vi "test_Template.vi"(8 "error in":errorcluster, 9 "tear down connection":bool, 10 "set-up a connection":bool, 11 "device selection":enum16{"monochromator", "CCD", "SCD"}(ring)) -> (0 "error out":errorcluster)   [LabVIEW 2023]
uses:
  Source/Classes/CCD/CCD.lvclass
  <vilib>/addons/_JKI Toolkits/Caraya/classes/Assert/Assert Not Error.vi
  <vilib>/addons/_JKI Toolkits/Caraya/classes/Assert/Assert Equal Value_Variant.vi
  Source/Classes/GenericDevice/GenericDevice.lvclass
  <vilib>/addons/_JKI Toolkits/Caraya/classes/Test/Test.lvclass
  <vilib>/addons/_JKI Toolkits/Caraya/classes/Assert/Assert.lvclass
panel:
  # "Connector Pane"
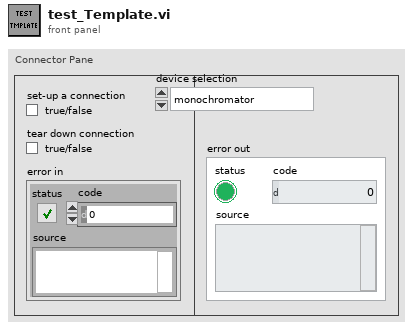
[diagram p1: front panel]
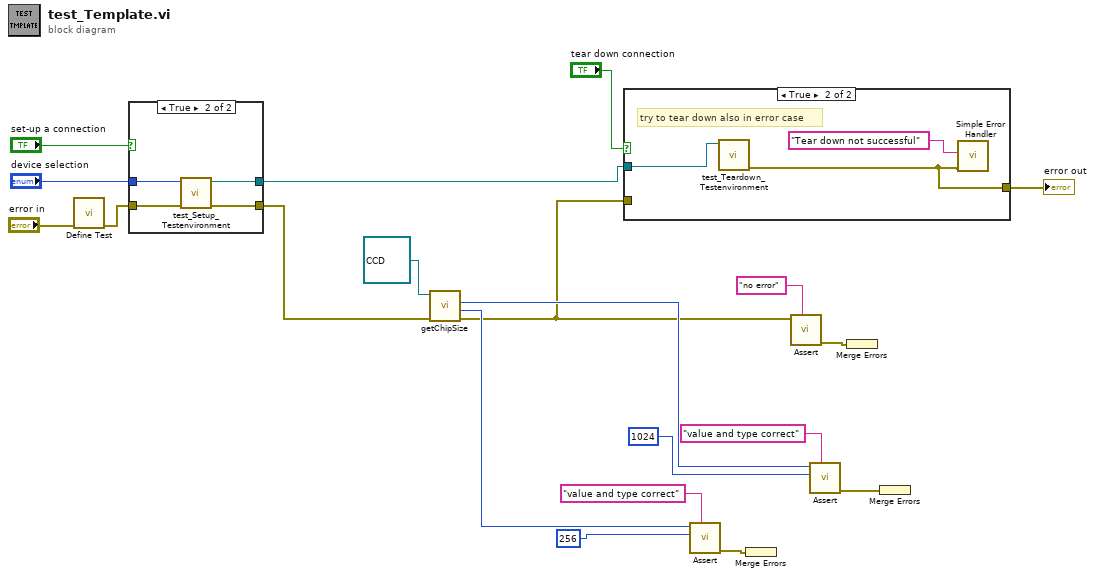
[diagram p0: block diagram]
diagram:
  n1 = call <vilib>:"Define Test.vi"("error in (no error)"="error in") -> ("error out"=w4:errorcluster)  [unwired: 9 in, 1 out]
  n2 = case shown="True" "set-up a connection" {
    tunnel: w4 -> [w21 w25]
    tunnel: [w21 w24] -> w6
    tunnel: "device selection" -> [_ w23]
    tunnel: [_ w22] -> w2
    frame False {
    }
    frame True {
      n3 = call "test_Setup_Testenvironment.vi"("error in"=w25, "device selection"=w23) -> ("error out"=w24:errorcluster, "GenericDevice.lvclass"=w22:refnum<class "GenericDevice.lvclass">)  [unwired: 7 in, 1 out]
    }
  }
  n4 = call-dynamic "getChipSize.vi"("error in (no error)"=w6, "CCD in"=refnum<class "CCD.lvclass"> refnum) -> ("error out"=w1:errorcluster, "chip size, y"=w7:i32, "chip size, x"=w15:i32)  [unwired: 6 in, 1 out]
  n5 = case shown="True" "tear down connection" {
    tunnel: w2 -> [_ w27]
    tunnel: [_ w26] -> w3
    tunnel: w1 -> [_ _]
    frame False {
    }
    frame True {
      # "try to tear down also in error case"
      n6 = call "test_Teardown_Testenvironment.vi"("GenericDevice.lvclass"=w27) -> ("error out"=w26:errorcluster)  [unwired: 9 in, 1 out]
      n7 = call <vilib>:"Simple Error Handler.vi"("error source (\" \")"="Tear down not successful" ("error source (\" \")"), "error in (no error)"=w26) -> ()  [unwired: 3 in, 5 out]
    }
  }
  "error out" <- w3
  n8 = call-poly <vilib>:"Assert.vi"("Label"="value and type correct" ("Label (VI Title)"), "Y"=256, "X"=w7) -> ("error out"=w11:errorcluster)  [unwired: 7 in, 1 out]
  n9 = Merge Errors(w11) -> ()  [unwired: 1 out]
  n10 = call-poly <vilib>:"Assert.vi"("Label"="no error" ("Label (VI Title)"), "Not Error?"=w1) -> ("error out"=w13:errorcluster)  [unwired: 8 in, 1 out]
  n11 = call-poly <vilib>:"Assert.vi"("Label"="value and type correct" ("Label (VI Title)"), "Y"=1024, "X"=w15) -> ("error out"=w17:errorcluster)  [unwired: 7 in, 1 out]
  n12 = Merge Errors(w13) -> ()  [unwired: 1 out]
  n13 = Merge Errors(w17) -> ()  [unwired: 1 out]
